vi "SSL_Get_Lib_Paths.vi"(8 "error in (no error)":errorcluster) -> (0 "error out":errorcluster, 2 "NIssleay":path)   [LabVIEW 2016, in "AWS_IoT.lvlib"]
doc: "Get path to NIssleay on each platform.\n\nMIT License\n\nCopyright (c) 2016 Indie-Energy\n\nPermission is hereby granted, free of charge, to any person obtaining a copy\nof this software and associated documentation files (the \"Software\"), to deal\nin the Software without restriction, including without limitation the rights\nto use, copy, modify, merge, publish, distribute, sublicense, and/or sell\ncopies of the Software, and to permit persons to whom the Software is\nfurnished to do so, subject to the following conditions:\n\nThe above copyright notice and this permission notice shall be included in all\ncopies or substantial portions of the Software.\n\nTHE SOFTWARE IS PROVIDED \"AS IS\", WITHOUT WARRANTY OF ANY KIND, EXPRESS OR\nIMPLIED, INCLUDING BUT NOT LIMITED TO THE WARRANTIES OF MERCHANTABILITY,\nFITNESS FOR A PARTICULAR PURPOSE AND NONINFRINGEMENT. IN NO EVENT SHALL THE\nAUTHORS OR COPYRIGHT HOLDERS BE LIABLE FOR ANY CLAIM, DAMAGES OR OTHER\nLIABILITY, WHETHER IN AN ACTION OF CONTRACT, TORT OR OTHERWISE, ARISING FROM,\nOUT OF OR IN CONNECTION WITH THE SOFTWARE OR THE USE OR OTHER DEALINGS IN THE\nSOFTWARE."
uses:
  AWS_IoT.lvlib
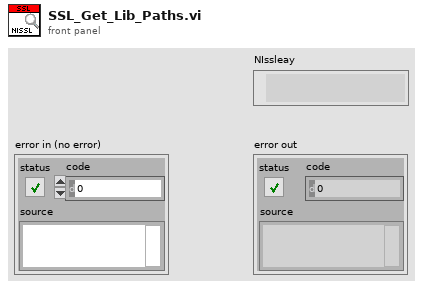
[diagram p1: front panel]
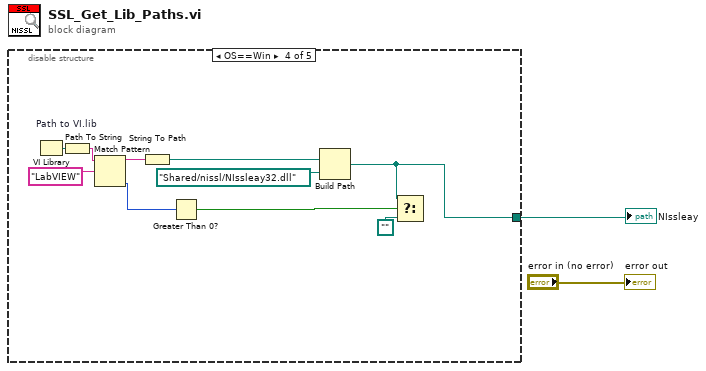
[diagram p0: block diagram]
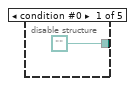
[diagram p2: hidden frame]
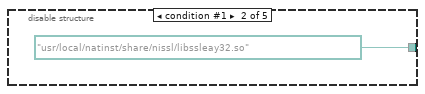
[diagram p3: hidden frame]
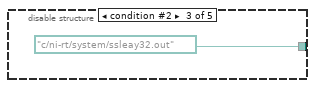
[diagram p4: hidden frame]
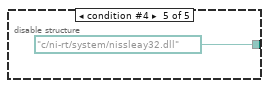
[diagram p5: hidden frame]
diagram:
  n1 = disable-structure shown="OS==Win" {
    disable-tunnel: [path "" path "/usr/local/natinst/share/nissl/libssleay32.so" ("SSL library path") path "c:/ni-rt/system/ssleay32.out" ("SSL library path") w8 path "c:/ni-rt/system/nissleay32.dll" ("SSL library path")] -> w2
    frame condition #0 {
    }
    frame condition #1 {
    }
    frame condition #2 {
    }
    frame condition #3 (active) {
      n2 = VI Library "Path to VI.lib"() -> (path=w13:path)
      n3 = Path To String(path=w13) -> (string=w14:string)
      n4 = Match Pattern(string=w14, regular expression="LabVIEW") -> (before substring=w12:string, offset past match=w11:i32)  [unwired: 1 in, 2 out]
      n5 = String To Path(string=w12) -> (path=w10:path)
      n6 = Greater Than 0?(x=w11) -> (x > 0?=w6:bool)
      n7 = Build Path(base path=w10, name or relative path=path "Shared/nissl/NIssleay32.dll" ("SSL library path")) -> (appended path=w8:path)
      n8 = Select(t=w8, s=w6, f=path "") -> ()  [unwired: 1 out]
    }
    frame condition #4 {
    }
  }
  "NIssleay" <- w2
  "error out" <- "error in (no error)"
